vi "Get Defualt JSON Param Documentation.vi"(8 "error in (no error)":errorcluster, 10 "request cluster":variant) -> (0 "error out":errorcluster, 2 "<JSON> Request Documentation":string)   [LabVIEW 2019, in "Help.lvclass"]
uses:
  Help.lvclass
  46988592-c207-47b7-8b61-3fcb2b203627.vi
  <vilib>/JDP Science/JSONtext/Variant to JSON Text.vi
  <vilib>/JDP Science/JSONtext/LVClass Serializer/JSONtext LVClass Serializer.lvclass
  <vilib>/JDP Science/JSONtext/JSONtext.lvlib
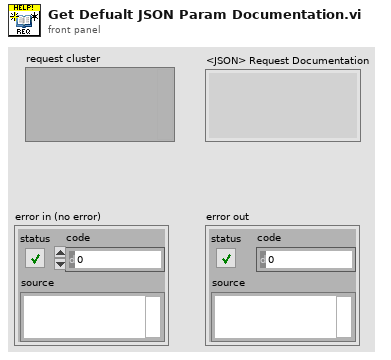
[diagram p1: front panel]
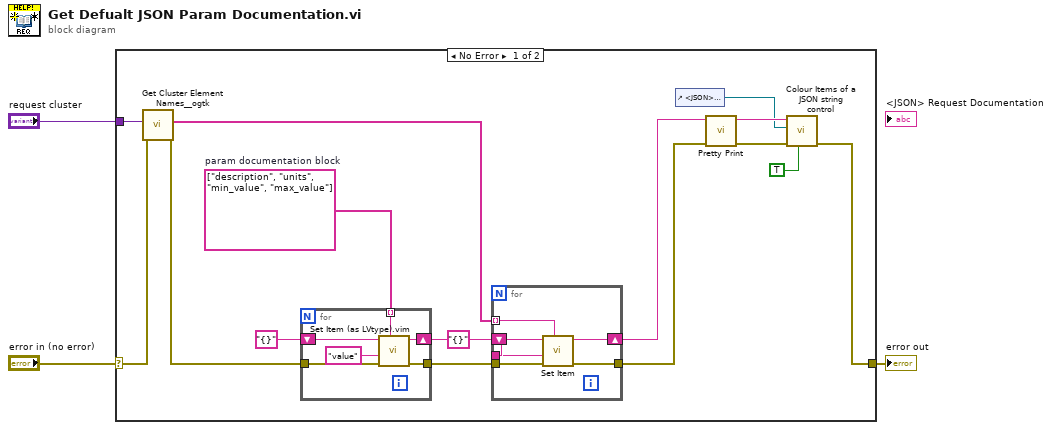
[diagram p0: block diagram]
diagram:
  n1 = case shown="No Error" "error in (no error)" {
    selector: "error in (no error)" -> [w11 w32]
    tunnel: "request cluster" -> [w19 _]
    tunnel: [w4 w32] -> w1
    frame No Error {
      w13 = string[] ["description", "units", "min_value", "max_value"]  # param documentation block
      n2 = call <userlib>:"Get Cluster Element Names__ogtk.vi"("error in (no error)"=w11, "Cluster"=w19) -> ("error out"=w12:errorcluster, "Element Names"=w15:string[])  [unwired: 8 in]
      n3 = for {
        tunnel: w13 -> [w30] mode=indexing
        shift-right: [w29] -> w17
        shift-left: "{}" ("JSON") -> [w31]
        tunnel: [w28] -> w16
        tunnel: w12 -> [w26]
        n4 = call "Set Item (as LVtype).vim"("$Path or Item Name"=w30, "error in (no error)"=w26, "Anything"="value", "JSON"=w31) -> ("error out"=w28:errorcluster, "<JSON>"=w29:string)  [unwired: 4 in, 1 out]
      }
      n5 = for {
        shift-right: [w24] -> w7
        shift-left: "{}" ("JSON") -> [w25]
        tunnel: [w23] -> w5
        tunnel: w17 -> [w22]
        tunnel: w15 -> [w21] mode=indexing
        tunnel: w16 -> [w20]
        n6 = call <vilib>:"Set Item.vi"("$Path or Item Name"=w21, "error in (no error)"=w20, "JSON to Insert"=w22, "JSON"=w25) -> ("error out"=w23:errorcluster, "<JSON>"=w24:string)  [unwired: 4 in, 1 out]
      }
      n7 = control-ref of="<JSON> Request Documentation"() -> (w6:refnum<vi>)
      n8 = call <vilib>:"Pretty Print.vi"("error in (no error)"=w5, "JSON"=w7) -> ("error out"=w9:errorcluster, "<JSON>"=w8:string)  [unwired: 7 in, 1 out]
      n9 = call <vilib>:"Colour Items of a JSON string control.vi"("Defer Panel Updates"=TRUE, "error in (no error)"=w9, "String Control"=w6, "JSON"=w8) -> ("error out"=w4:errorcluster)  [unwired: 7 in]
    }
    frame Error {
    }
  }
  "error out" <- w1
